vi "Stack Temp HMI Screen Dev (page 1).vi"() -> ()   [LabVIEW 2019]
uses:
  <vilib>/10X Engineering/Custom Flat Buttons UI Controls/Buttons/sign out/Sign out 1.ctl
  <vilib>/10X Engineering/Custom Flat Buttons UI Controls/Buttons/add/Add 2.ctl
  <vilib>/10X Engineering/Custom Flat Buttons UI Controls/Buttons/remove/Remove 2.ctl
  <vilib>/10X Engineering/Custom Flat Buttons UI Controls/Custom Flat Buttons UI Controls.lvlib
panel:
  out "remove 3":T1
  out "remove 2":T1
  out "remove":T1
  out "Add 3":T2
  out "Add 2":T2
  out "Add":T2
  out "sign out":T3
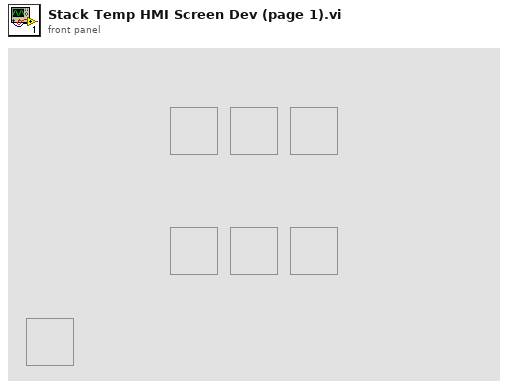
[diagram p1: front panel]
types:
  T1 = typedef "Custom Flat Buttons UI Controls.lvlib/Remove 2.ctl" = bool
  T2 = typedef "Custom Flat Buttons UI Controls.lvlib/Add 2.ctl" = bool
  T3 = typedef "Custom Flat Buttons UI Controls.lvlib/Sign out 1.ctl" = bool
  T4 = typedef "imagedata.ctl" = cluster{"image type":i32, "image depth":i32, "image":u8[], "mask":u8[], "colors":u32[], "Rectangle":cluster{"left":i16, "top":i16, "right":i16, "bottom":i16}}
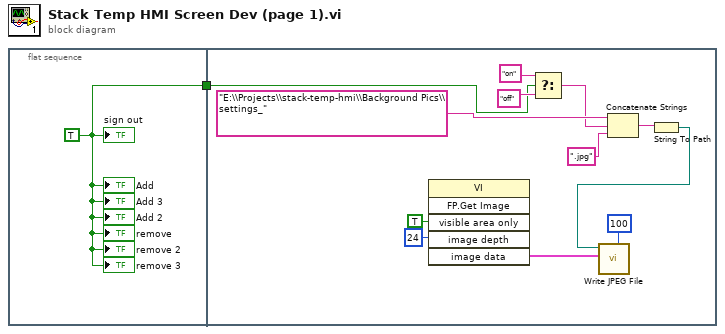
[diagram p0: block diagram]
diagram:
  n1 = flat-sequence {
    tunnel: [w2] -> w1
    tunnel: w1 -> [w4]
    frame #0 {
      w2 = TRUE ("s")
      "sign out" <- w2
      "Add" <- w2
      "Add 2" <- w2
      "Add 3" <- w2
      "remove" <- w2
      "remove 2" <- w2
      "remove 3" <- w2
    }
    frame #1 {
      n2 = invoke class="VI" method="FP.Get Image"("visible area only"=TRUE ("Visible Area Only"), "image depth"=24 ("Image Depth")) -> ("image data"=w13:T4)  [unwired: 4 in, 5 out]
      n3 = Select(t="on" ("string"), s=w4, f="off" ("string")) -> (s? t:f=w3:string)
      n4 = Concatenate Strings("E:\\Projects\\stack-temp-hmi\\Background Pics\\settings_", w3, ".jpg" ("string")) -> (w8:string)
      n5 = String To Path(string=w8) -> (path=w10:path)
      n6 = call <vilib>:"Write JPEG File.vi"("quality (80)"=100, "image data"=w13, "path to JPEG file"=w10) -> ()  [unwired: 7 in, 2 out]
    }
  }
